vi "stageMoveTo.vi"() -> ()   [LabVIEW 2017]
panel:
  in  "stop":bool
  in  "position (um)":dbl
  # "Move stage to absolute position"
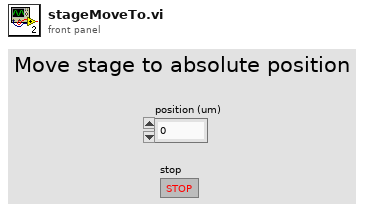
[diagram p1: front panel]
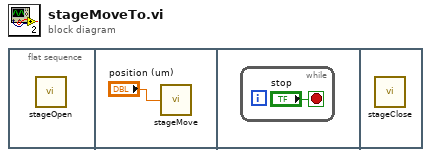
[diagram p0: block diagram]
diagram:
  n1 = flat-sequence {
    frame #0 {
      n2 = call "stageOpen.vi"() -> ()  [unwired: 2 out]
    }
    frame #1 {
      n3 = call "stageMove.vi"("position (um)"="position (um)") -> ()  [unwired: 2 out]
    }
    frame #2 {
      n4 = while {
        stop <- "stop" stop-if-true
      }
    }
    frame #3 {
      n5 = call "stageClose.vi"() -> ()  [unwired: 1 out]
    }
  }
